vi "Contour Line (Array).vi"(8 "Heights":dbl[](array[numeric]), 9 "Z":dbl[][](array[numeric]), 10 "Y":dbl[](array[numeric]), 11 "X":dbl[](array[numeric])) -> (0 "error":i32, 2 "Contour Line":T1[](array[typedef]), 3 "Contour Graph":cluster{dbl[], dbl[]}[](graph))   [LabVIEW 2020, in "NI_AAL_Geometry.lvlib"]
doc: "Calculates and returns the contour lines of a surface and the contour graph."
uses:
  <vilib>/Analysis/NI_AAL_Geometry.lvlib
  <vilib>/Analysis/geometry.llb/Contour Lines Control.ctl
  <vilib>/Analysis/geometry.llb/Contour Line Segment.ctl
  <vilib>/gmath/interp.llb/Create Mesh Grid (2D) (x,y arrays).vi
  <vilib>/gmath/NI_Gmath.lvlib
panel:
  # "Contour Line"
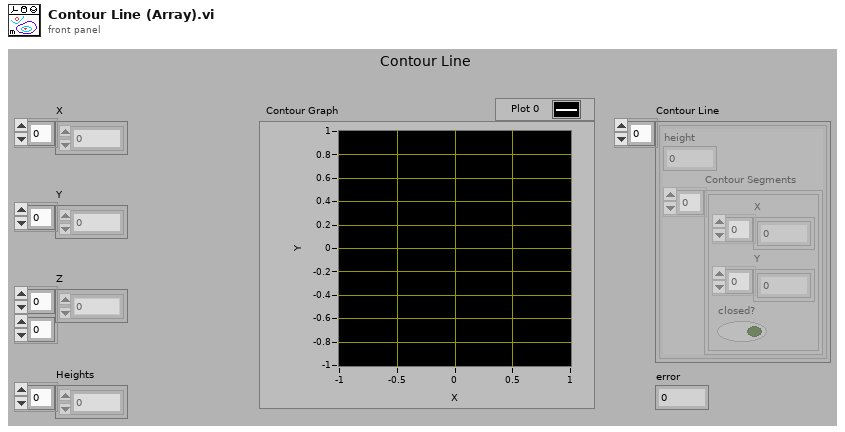
[diagram p1: front panel]
types:
  T1 = typedef "NI_AAL_Geometry.lvlib/Contour Lines Control.ctl" = cluster{"height":dbl, "Contour Segments":T2[]}
  T2 = typedef "NI_AAL_Geometry.lvlib/Contour Line Segment.ctl" = cluster{"X":dbl[], "Y":dbl[], "closed?":bool}
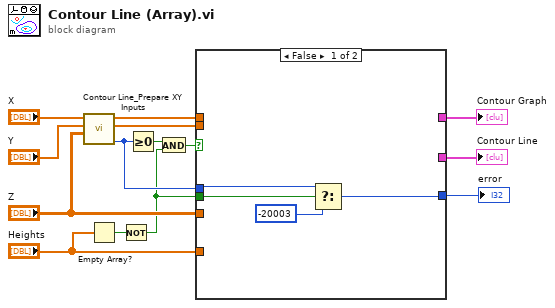
[diagram p0: block diagram]
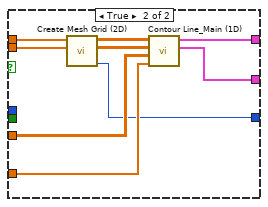
[diagram p2: hidden frame]
diagram:
  n1 = call <vilib>:"Contour Line_Prepare XY Inputs.vi"("Z In"="Z", "Y In"="Y", "X In"="X") -> ("error"=w7:i32, "Y Out"=w8:dbl[], "X Out"=w9:dbl[])  [unwired: 6 in]
  n2 = Empty Array?(array="Heights") -> (empty?=w3:bool)
  n3 = Not(x=w3) -> (.not. x?=w2:bool)
  n4 = Greater Or Equal To 0?(x=w7) -> (x >= 0?=w4:bool)
  n5 = And(x=w4, y=w2) -> (x .and. y?=w1:bool)
  n6 = case shown="False" w1 {
    tunnel: "Heights" -> [_ w27]
    tunnel: [_ w26] -> w14
    tunnel: [_ w25] -> w13
    tunnel: "Z" -> [_ w24]
    tunnel: w9 -> [_ w23]
    tunnel: w8 -> [_ w22]
    tunnel: w7 -> [w16 _]
    tunnel: [w17 w19] -> w6
    tunnel: w2 -> [w18 _]
    frame False {
      n7 = Select(t=w16, s=w18, f=-20003) -> (s? t:f=w17:i32)
    }
    frame True {
      n8 = call-poly <vilib>:"Create Mesh Grid (2D).vi"("y domain"=w22, "x domain"=w23) -> ("error"=w19:i32, "Y"=w20:dbl[][], "X"=w21:dbl[][])  [unwired: 7 in]
      n9 = call <vilib>:"Contour Line_Main (1D).vi"("Heights"=w27, "Z"=w24, "Y"=w20, "X"=w21) -> ("Contour Line"=w25:T1[], "Contour Graph"=w26:cluster{dbl[], dbl[]}[])  [unwired: 6 in]
    }
  }
  "error" <- w6
  "Contour Line" <- w13
  "Contour Graph" <- w14
